vi "Add Zenoh Error.vi"(8 "error in (no error)":errorcluster, 9 "String to Append":string, 10 "Error":T1, 11 "Insert Error":bool=TRUE) -> (0 "error out":errorcluster)   [LabVIEW 2021, in "Zenoh.lvclass"]
uses:
  Zenoh.lvclass
  typedef/Zenoh Errors.ctl
  Zenoh.lvclass/Zenoh.ctl
  <vilib>/CIF Foundation/CIF Utilities/Errors/Errors_CIF_U.lvlib
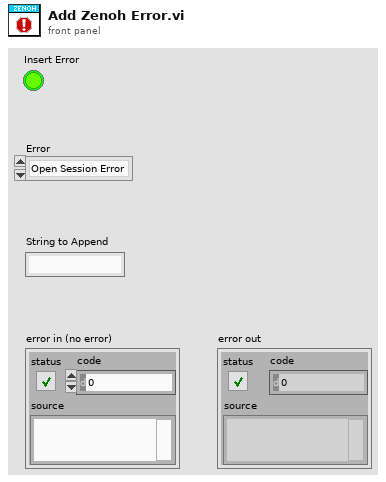
[diagram p1: front panel]
types:
  T1 = typedef "Zenoh.lvclass/Zenoh Errors.ctl" = enum16{"Open Session Error", "Open Subscription Error"}
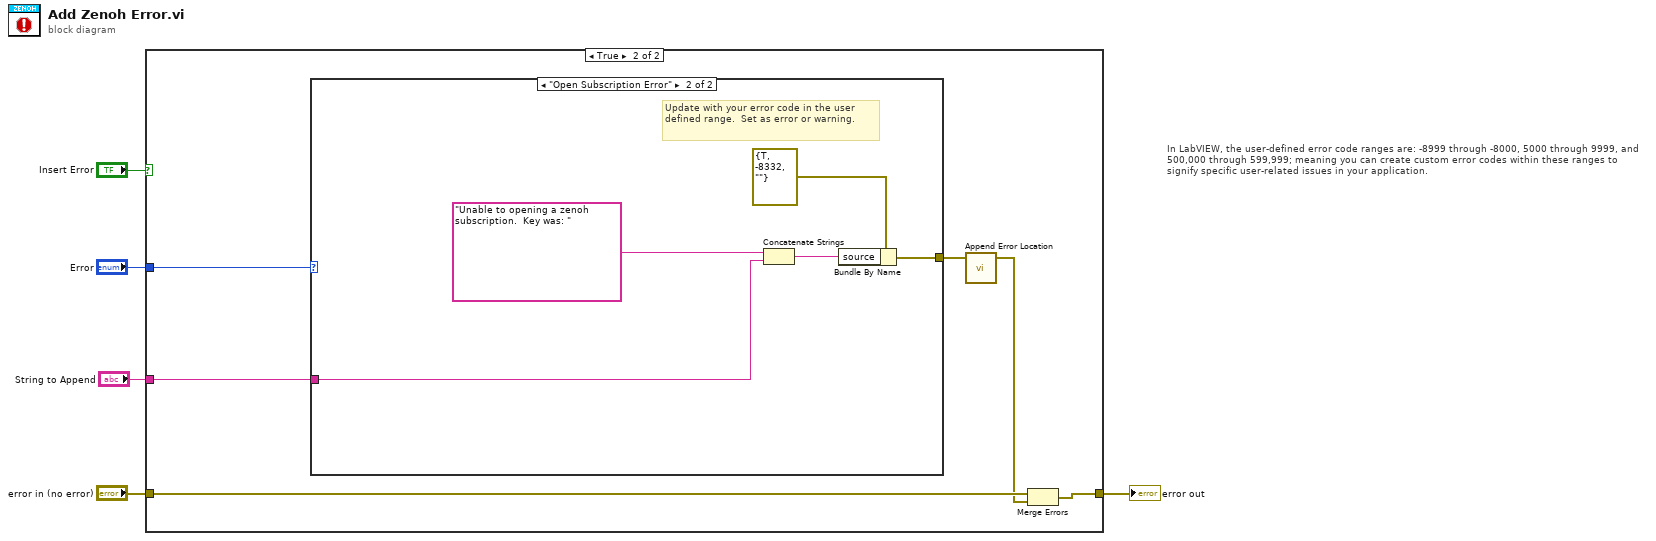
[diagram p0: block diagram]
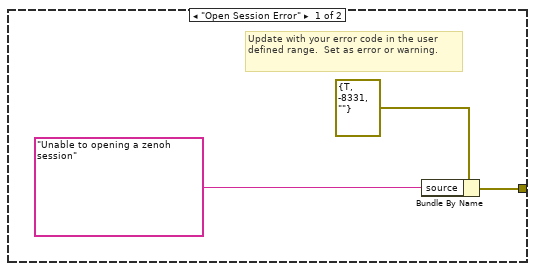
[diagram p3: hidden frame]
diagram:
  # "In LabVIEW, the user-defined error code ranges are: -8999 through -8000, 5000 through 9999, and 500,000 through 599,999; meaning you can create custom error codes within these ranges to signify specific user-related issues in your application."
  n1 = case shown="True" "Insert Error" {
    tunnel: [w6 w9] -> w4
    tunnel: "error in (no error)" -> [w6 w10]
    tunnel: "Error" -> [_ w12]
    tunnel: "String to Append" -> [_ w11]
    frame False {
    }
    frame True {
      n2 = case shown="\"Open Subscription Error\"" w12 {
        tunnel: w11 -> [_ w16]
        tunnel: [w14 w19] -> w8
        frame "Open Session Error" {
          # "Update with your error code in the user defined range.  Set as error or warning."
          n3 = Bundle By Name(cluster=errorcluster {"status"=TRUE, "code"=-8331, "source"=""} ("Invalid ID"), "source"="Unable to opening a zenoh session") -> (w14:errorcluster)
        }
        frame "Open Subscription Error" {
          # "Update with your error code in the user defined range.  Set as error or warning."
          n4 = Concatenate Strings("Unable to opening a zenoh subscription.  Key was: " ("source"), w16) -> (w17:string)
          n5 = Bundle By Name(cluster=errorcluster {"status"=TRUE, "code"=-8332, "source"=""} ("Invalid ID"), "source"=w17) -> (w19:errorcluster)
        }
      }
      n6 = call <vilib>:"Append Error Location.vi"("error in (no error)"=w8) -> ("error out"=w7:errorcluster)  [unwired: 4 in]
      n7 = Merge Errors(w10, w7) -> (w9:errorcluster)
    }
  }
  "error out" <- w4
